vi "ESP_Full_State_Test_TCP.vi"() -> ()   [LabVIEW 2021]
panel:
  out "error out":errorcluster
  in  "UDP Activate":bool
  out "output array":sgl[][](array[numeric])
  out "Waveform Chart 2":sgl[][](graph)
  in  "stop streaming":bool
  in  "Shut dowm":bool
  in  "Full state":bool
  in  "Stream":bool
  in  "Re-zero":bool
  out "Waveform Chart":sgl[](graph)
  out "Stream on?":string
  # "Sampling rate is 225 Hz, please use the Setup software to change the rate"
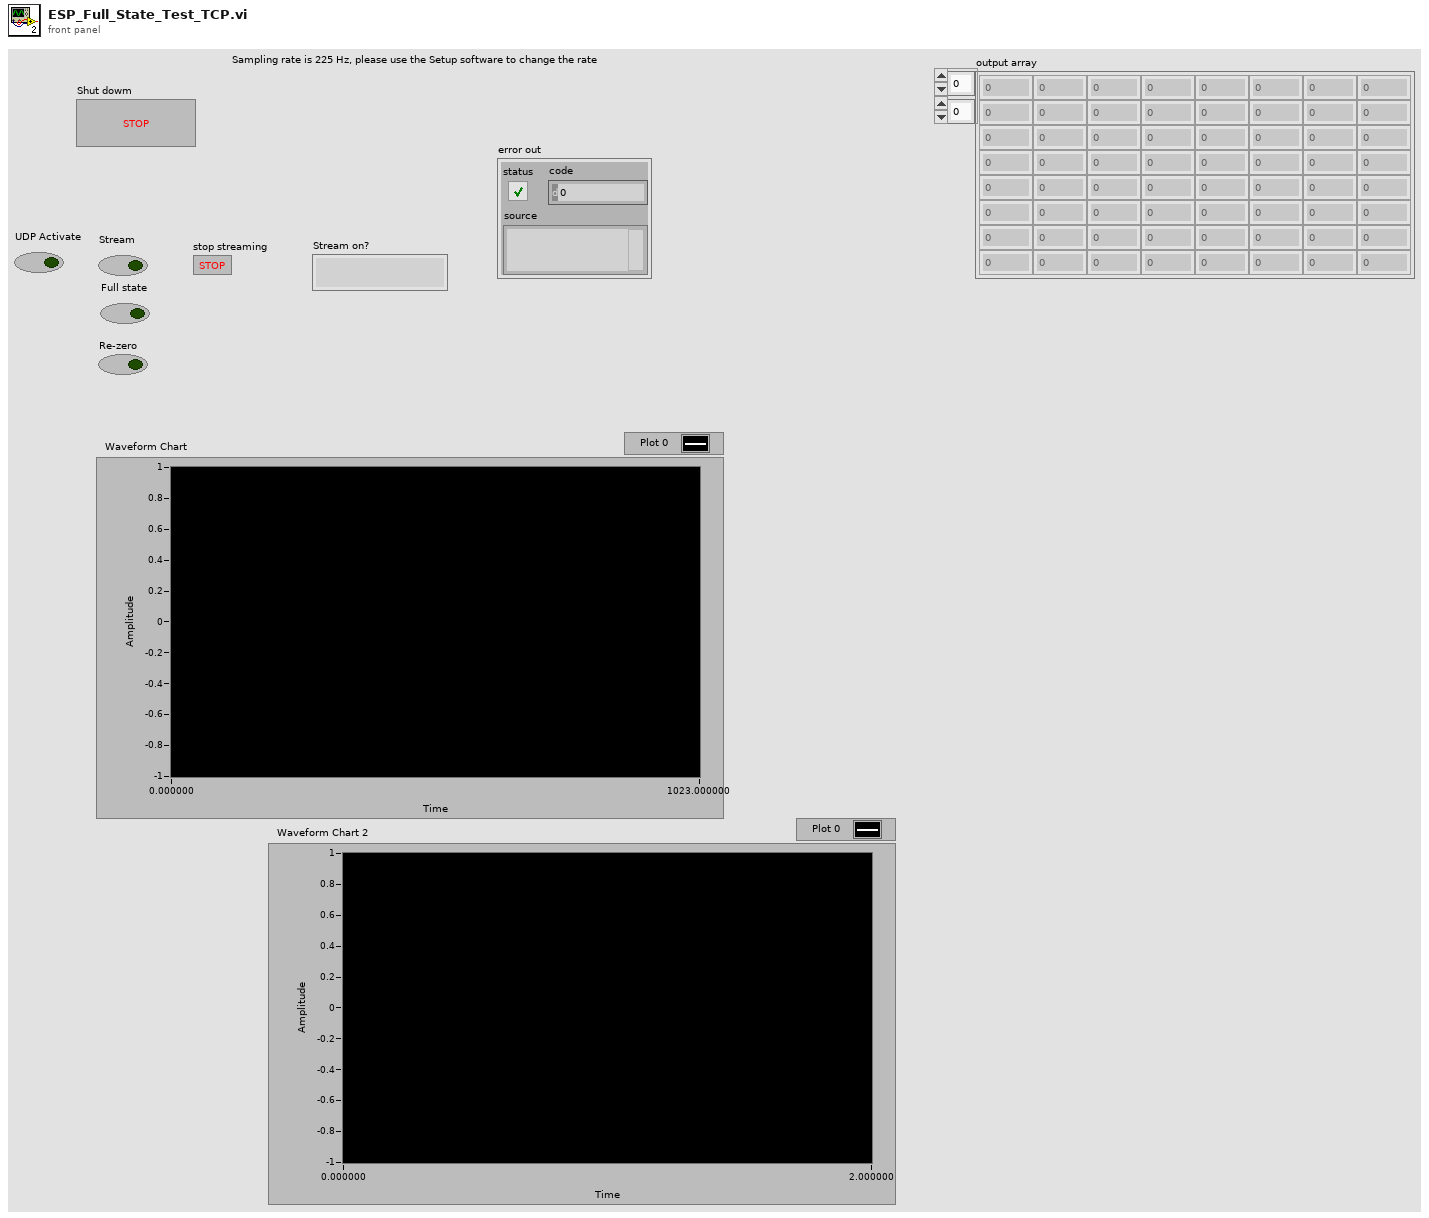
[diagram p1: front panel]
types:
  T1 = enum16{"Standard", "Buffered", "CRLF", "Immediate"}
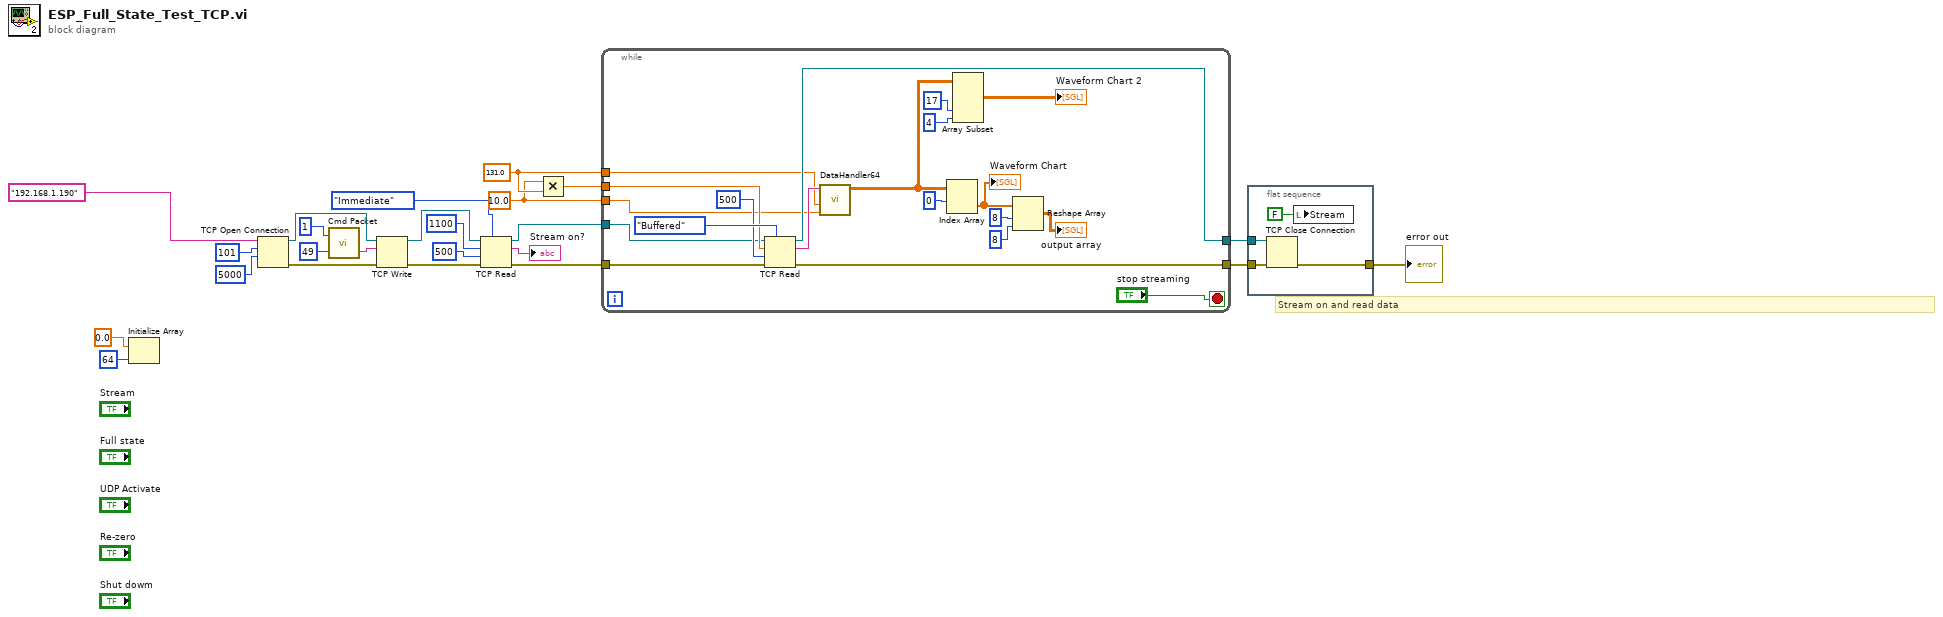
[diagram p0: block diagram]
diagram:
  w7 = 10.0 ("Sampling Rate")
  w8 = 131.0 ("y")
  # "Stream on and read data"
  n1 = Initialize Array(0.0, 64) -> ()  [unwired: 1 out]
  n2 = TCP Open Connection(address="192.168.1.190", remote port or service name=u16 101 ("Port"), timeout ms (60000)=5000) -> (connection ID=w16:refnum<k5>, error out=w6:errorcluster)  [unwired: 2 in]
  n3 = call "Cmd Packet.vi"("Command Byte"=49 ("data in"), "Parameter Byte"=1 ("data in")) -> ("Command Packet Byte String"=w20:string)  [unwired: 1 out]
  n4 = TCP Write(connection ID=w16, data in=w20, error in (no error)=w6) -> (connection ID out=w18:refnum<k5>, error out=w5:errorcluster)  [unwired: 1 in, 1 out]
  n5 = TCP Read(connection ID=w18, bytes to read=1100, error in (no error)=w5, 7:T1."Immediate" ("mode (standard)"), 9:500 ("timeout ms (25000)")) -> (connection ID out=w21:refnum<k5>, data out=→"Stream on?":string, error out=w4:errorcluster)
  n6 = Multiply(x=w7, y=w8) -> (x*y=w17:dbl)
  n7 = while {
    tunnel: [w41] -> w22
    tunnel: w21 -> [w37]
    tunnel: w17 -> [w40]
    tunnel: w8 -> [w39]
    tunnel: w7 -> [w38]
    tunnel: w4 -> [w26]
    tunnel: [w25] -> w3
    stop <- "stop streaming" stop-if-true
    n8 = TCP Read(connection ID=w37, bytes to read=w40, error in (no error)=w26, 7:T1."Buffered" ("mode (standard)"), 9:500 ("timeout ms (25000)")) -> (connection ID out=w41:refnum<k5>, data out=w44:string, error out=w25:errorcluster)
    n9 = call "DataHandler64.vi"("Data Cycles Per Buffer"=w38, "Rx Packet Byte size"=w39, "data out"=w44) -> ("Data"=w27:sgl[][])  [unwired: 2 in, 4 out]
    n10 = Index Array(array=w27, index (row)=0 ("Channel")) -> (element=w29:sgl[])  [unwired: 1 in]
    "Waveform Chart" <- w29
    n11 = Array Subset(array=w27, index (col)=17 ("index"), length (col)=4 ("length")) -> (→"Waveform Chart 2":sgl[][])  [unwired: 2 in]
    n12 = Reshape Array(w29, 8 ("dimension size"), 8 ("dimension size")) -> (→"output array":sgl[][])
  }
  n13 = flat-sequence {
    tunnel: w22 -> [w47]
    tunnel: w3 -> [w46]
    tunnel: [w45] -> w2
    frame #0 {
      n14 = TCP Close Connection(connection ID=w47, error in (no error)=w46) -> (error out=w45:errorcluster)  [unwired: 1 in, 1 out]
      n15 = local write "Stream"(FALSE) -> ()
    }
  }
  "error out" <- w2
